vi "Display ListSelection.vi"(8 "error in (no error)":errorcluster, 10 "Visible(False)":bool, 11 "ListSelection in":refnum<class "ListSelection.lvclass">) -> (0 "error out":errorcluster, 3 "ListSelection out":refnum<class "ListSelection.lvclass">)   [LabVIEW 2015, in "Admin_Actor.lvlib" / "ListSelection.lvclass"]
uses:
  ListSelection.lvclass
  ListSelection.lvclass/ListSelection.ctl
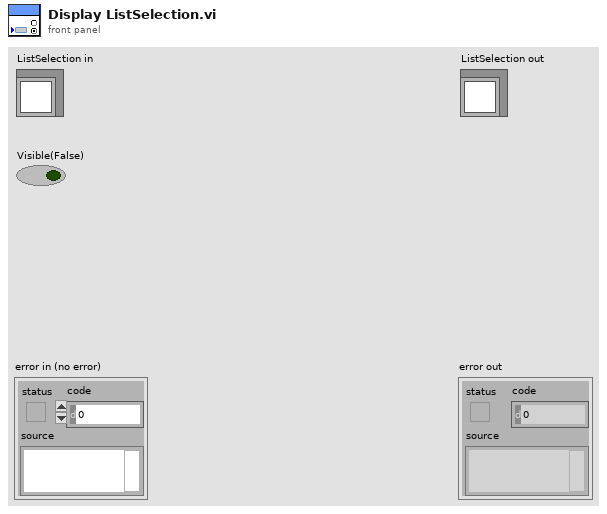
[diagram p1: front panel]
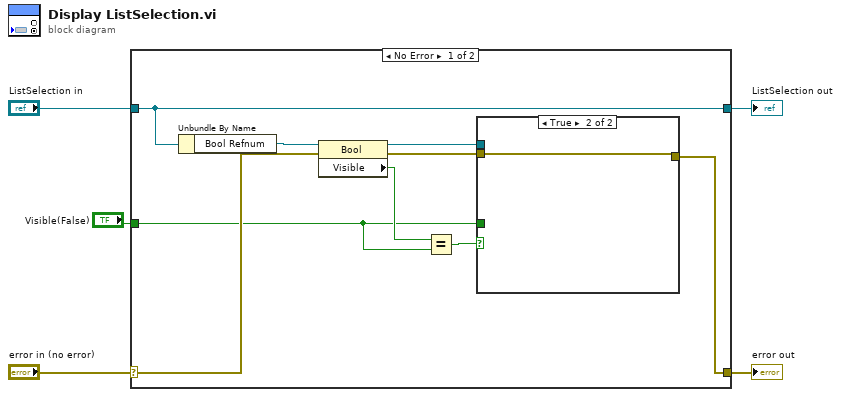
[diagram p0: block diagram]
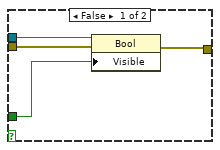
[diagram p2: hidden frame]
diagram:
  n1 = case shown="No Error" "error in (no error)" {
    selector: "error in (no error)" -> [w11 w21]
    tunnel: [w13 w21] -> w4
    tunnel: [w14 w20] -> w2
    tunnel: "ListSelection in" -> [w14 w20]
    tunnel: "Visible(False)" -> [w9 _]
    frame No Error {
      n2 = Unbundle By Name(w14) -> ("Bool Refnum"=w12:refnum<vi>)
      n3 = property class="Bool"(reference=w12, error in=w11) -> (reference out=w7:refnum<vi>, error out=w6:errorcluster, "Visible"=w10:bool)
      n4 = Equal?(x=w10, y=w9) -> (x = y?=w8:bool)
      n5 = case shown="True" w8 {
        tunnel: [w18 w19] -> w13
        tunnel: w9 -> [w17 _]
        tunnel: w7 -> [w15 _]
        tunnel: w6 -> [w16 w19]
        frame False {
          n6 = property class="Bool"(reference=w15, error in=w16, "Visible"=w17) -> (error out=w18:errorcluster)  [unwired: 1 out]
        }
        frame True {
        }
      }
    }
    frame Error {
    }
  }
  "error out" <- w4
  "ListSelection out" <- w2
